vi "relay_init.vi"() -> ()   [LabVIEW 2010]
uses:
  <vilib>/Instr/_visa.llb/VISA Configure Serial Port (Instr).vi
panel:
  in  "init?":bool=TRUE
  in  "VISA resource name":refnum<visa-resource-name>="ASRL2::INSTR"
  in  "error in":errorcluster
  in  "Port Configuration":T1={"baud rate (9600)"=9600, "data bits (8)"=8, "parity (0:none)"=enum."None", "stop bits (10: 1 bit)"=10, "flow control (0:none)"=0, "timeout (10sec)"=10000, "termination char\n(0xA = '\\n' = LF) "=10, "Enable Termination\nChar (T)"=TRUE} {"termination char\n(0xA = '\\n' = LF)" format="%.0x"; "flow control (0:none)" items=["None", "XON/XOFF", "RTS/CTS", "XON/XOFF & RTS/CTS", "DTR/DSR", "XON/XOFF & DTR/DSR"]; "stop bits (10: 1 bit)" items=["1.0"=10, "1.5"=15, "2.0"=20]; "data bits (8)" min=5 max=8 step=1}
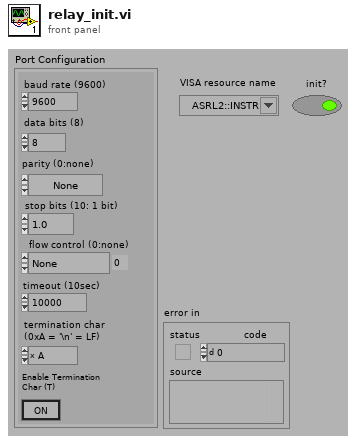
[diagram p1: front panel]
types:
  T1 = cluster{"baud rate (9600)":u32, "data bits (8)":u16, "parity (0:none)":enum16{"None", "Odd", "Even", "Mark", "Space"}, "stop bits (10: 1 bit)":u16, "flow control (0:none)":u16, "timeout (10sec)":u32, "termination char\n(0xA = '\\n' = LF) ":u8, "Enable Termination\nChar (T)":bool}
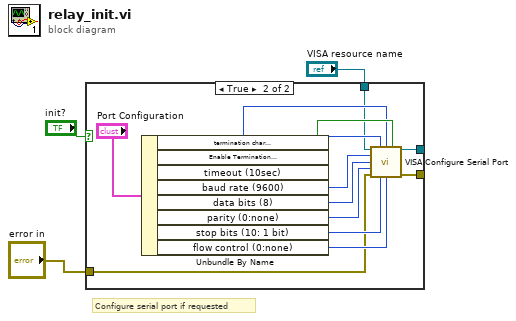
[diagram p0: block diagram]
diagram:
  # "Configure serial port if requested"
  n1 = case shown="True" "init?" {
    tunnel: [w4 w9] -> _
    tunnel: [w5 w8] -> _
    tunnel: "error in" -> [w5 w7]
    tunnel: "VISA resource name" -> [w4 w6]
    frame False {
    }
    frame True {
      n2 = Unbundle By Name("Port Configuration") -> ("termination char\n(0xA = '\\n' = LF)"=w10:u8, "Enable Termination\nChar (T)"=w11:bool, "timeout (10sec)"=w12:u32, "baud rate (9600)"=w17:u32, "data bits (8)"=w16:u16, "parity (0:none)"=w15:enum16{"None", "Odd", "Even", "Mark", "Space"}, "stop bits (10: 1 bit)"=w14:u16, "flow control (0:none)"=w13:u16)
      n3 = call-poly "VISA Configure Serial Port"("VISA resource name"=w6, "timeout (10sec)"=w12, "termination char\n(0xA = '\\n' = LF)"=w10, "Enable Termination\nChar (T)"=w11, "baud rate (9600)"=w17, "data bits (8)"=w16, "parity (0:none)"=w15, "error in (no error)"=w7, "stop bits (10: 1 bit)"=w14, "flow control (0:none)"=w13) -> ("VISA resource name out"=w9:refnum<visa-resource-name>, "error out"=w8:errorcluster)  [unwired: 4 in]
    }
  }
